vi "Translate.vi"(0 "reference":refnum<class "SegmentedLineEdge.lvclass">, 1 "dx":dbl format="%.2f", 2 "dy":dbl format="%.2f", 3 "StartEndNode":refnum<class "AbstractNode.lvclass">, 5 "error in (no error)":errorcluster) -> (14 "reference out":refnum<class "SegmentedLineEdge.lvclass">, 19 "error out":errorcluster)   [LabVIEW 2020, in "SegmentedLineEdge.lvclass"]
doc: "Translate"
uses:
  <resource>/Framework/Providers/Open_GDS/UML/SegmentedLineEdge_class/SegmentedLineEdge.lvclass
  <resource>/Framework/Providers/Open_GDS/UML/AbstractNode_class/AbstractNode.lvclass
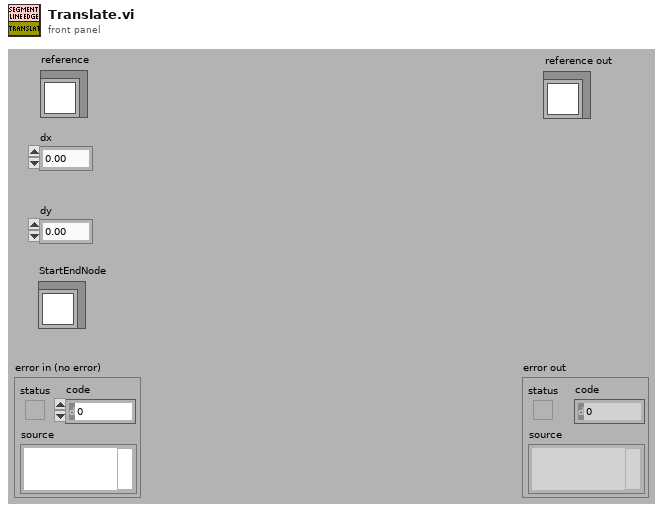
[diagram p1: front panel]
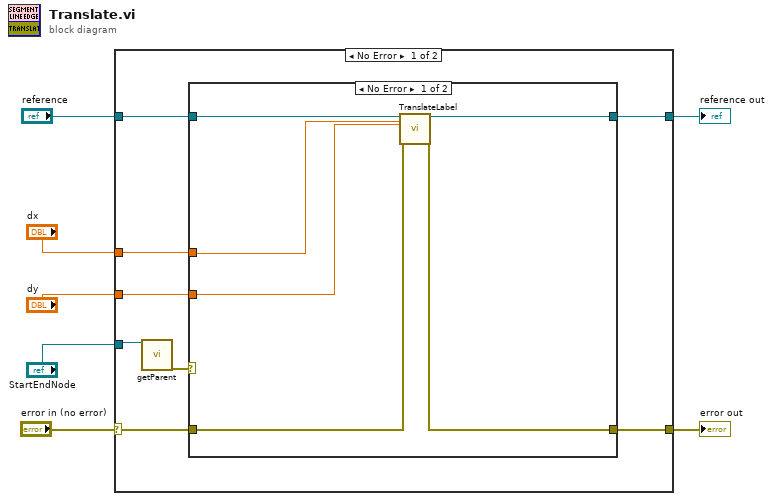
[diagram p0: block diagram]
diagram:
  n1 = case shown="No Error" "error in (no error)" {
    selector: "error in (no error)" -> [w14 w24]
    tunnel: "reference" -> [w15 w25]
    tunnel: [w10 w24] -> w5
    tunnel: [w11 w25] -> w4
    tunnel: "StartEndNode" -> [w9 _]
    tunnel: "dy" -> [w13 _]
    tunnel: "dx" -> [w12 _]
    frame No Error {
      n2 = call-dynamic "getParent.vi"("reference"=w9) -> ("error out"=w8:errorcluster)  [unwired: 14 in, 4 out]
      n3 = case shown="No Error" w8 {
        tunnel: w14 -> [w18 w23]
        tunnel: w15 -> [w21 w22]
        tunnel: [w17 w23] -> w10
        tunnel: w12 -> [w20 _]
        tunnel: w13 -> [w19 _]
        tunnel: [w16 w22] -> w11
        frame No Error {
          n4 = call <resource>:"TranslateLabel.vi"("reference"=w21, "dx"=w20, "dy"=w19, "error in (no error)"=w18) -> ("reference out"=w16:refnum<class "SegmentedLineEdge.lvclass">, "error out"=w17:errorcluster)  [unwired: 1 in, 13 out]
        }
        frame Error {
        }
      }
    }
    frame Error {
    }
  }
  "reference out" <- w4
  "error out" <- w5
